vi "Update_Referenced.vi"(8 "error in (no error)":errorcluster, 9 "Referenced?":bool, 10 "PV-URL":string, 11 "CS++Motor in":refnum<class "CS++Motor.lvclass">) -> (0 "error out":errorcluster, 3 "CS++Motor out":refnum<class "CS++Motor.lvclass">)   [LabVIEW 2015, in "CS++Motor.lvlib" / "CS++Motor.lvclass"]
doc: "This VI is executed via the corresponding Monitor Actor and delivers the information wether an axis is referenced or not."
uses:
  CS++Motor.lvclass
  CS++Motor.lvclass/CS++Motor.ctl
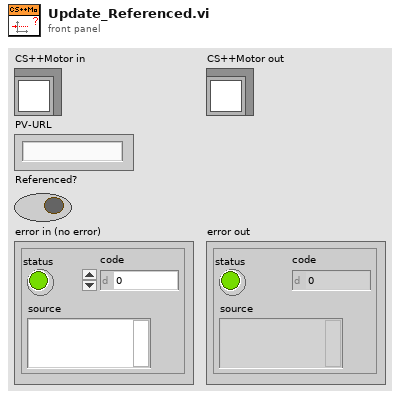
[diagram p1: front panel]
types:
  T1 = cluster{"Update-Msg Name":string, "Update-Msg URLs":string[]}[]
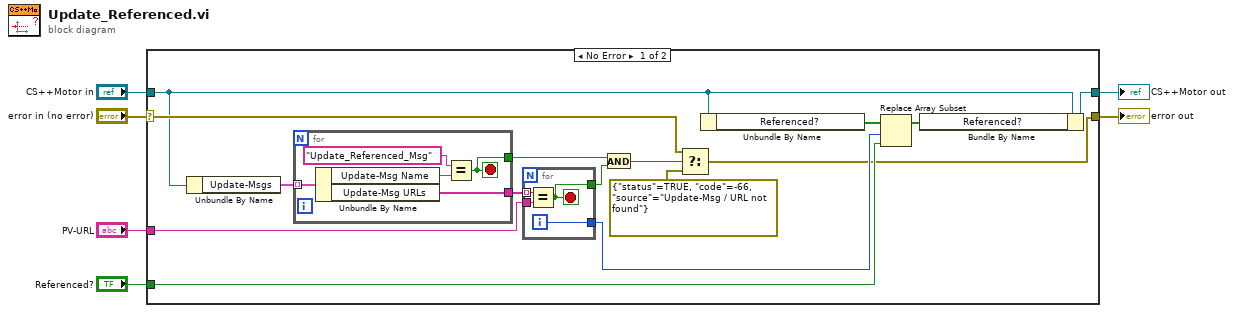
[diagram p0: block diagram]
diagram:
  n1 = case shown="No Error" "error in (no error)" {
    selector: "error in (no error)" -> [w14 w32]
    tunnel: [w7 w32] -> w5
    tunnel: [w12 w31] -> w3
    tunnel: "CS++Motor in" -> [w13 w31]
    tunnel: "Referenced?" -> [w9 _]
    tunnel: "PV-URL" -> [w15 _]
    frame No Error {
      n2 = Unbundle By Name(w13) -> ("Update-Msgs"=w16:T1)
      n3 = for {
        tunnel: w16 -> [w30] mode=indexing
        tunnel: [w27] -> w21
        tunnel: [w26] -> w20
        stop <- w26 stop-if-true
        n4 = Unbundle By Name(w30) -> ("Update-Msg Name"=w29:string, "Update-Msg URLs"=w27:string[])
        n5 = Equal?(x="Update_Referenced_Msg", y=w29) -> (x = y?=w26:bool)
      }
      n6 = for {
        tunnel: w21 -> [w25] mode=indexing
        tunnel: w15 -> [w24]
        tunnel: [w23] -> w19
        tunnel: [w22] -> w8
        i -> [w22]
        stop <- w23 stop-if-true
        n7 = Equal?(x=w25, y=w24) -> (x = y?=w23:bool)
      }
      n8 = And(x=w20, y=w19) -> (x .and. y?=w18:bool)
      n9 = Select(t=w14, s=w18, f=errorcluster {"status"=TRUE, "code"=-66, "source"="Update-Msg / URL not found"}) -> (s? t:f=w7:errorcluster)
      n10 = Unbundle By Name(w13) -> ("Referenced?"=w11:bool[])
      n11 = Replace Array Subset(array=w11, new element=w9, index=w8) -> (w10:bool[])
      n12 = Bundle By Name(cluster=w13, "Referenced?"=w10) -> (w12:refnum<class "CS++Motor.lvclass">)
    }
    frame Error {
    }
  }
  "error out" <- w5
  "CS++Motor out" <- w3
